vi "H5Tdetect_class.vi"(6 "error in (no error)":errorcluster, 8 "Class":T1 items=["H5T_NO_CLASS"=-1, "H5T_INTEGER"=0, "H5T_FLOAT"=1, "H5T_TIME"=2, "H5T_STRING"=3, "H5T_BITFIELD"=4, "H5T_OPAQUE"=5, "H5T_COMPOUND"=6, "H5T_REFERENCE"=7, "H5T_ENUM"=8, "H5T_VLEN"=9, "H5T_ARRAY"=10], 9 "HDF5 Type Ref":T2) -> (0 "error out":errorcluster, 2 "Detected":bool, 3 "HDF5 Type Ref out":T2)   [LabVIEW 2017]
doc: "Determines whether a datatype contains any datatypes of the \n given datatype class."
uses:
  <vilib>/UPVI/lvhdf5/library.llb/HDF5 Ref.ctl
  <vilib>/UPVI/lvhdf5/datatype.llb/H5T_class_t.ctl
  <vilib>/UPVI/lvhdf5/hdf5.dll
panel:
  # "LVHDF5 Toolkit\nCopyright (c) 2005-2013 by Jason D. Sommerville\nCopyright (c) 2014 by UPVI, LLC.\n\nThis use and distribution of this file is governed by the terms found in \nLICENSE.txt distributed with this toolkit and installed at\n <user.lib>\\_lvhdf5\\LICENSE.txt"
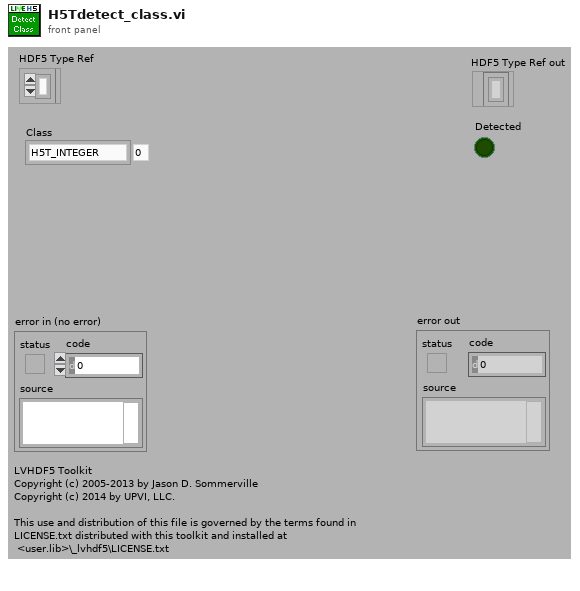
[diagram p1: front panel]
types:
  T1 = typedef "H5T_class_t.ctl" = i32
  T2 = typedef "HDF5 Ref.ctl" = refnum<k1>
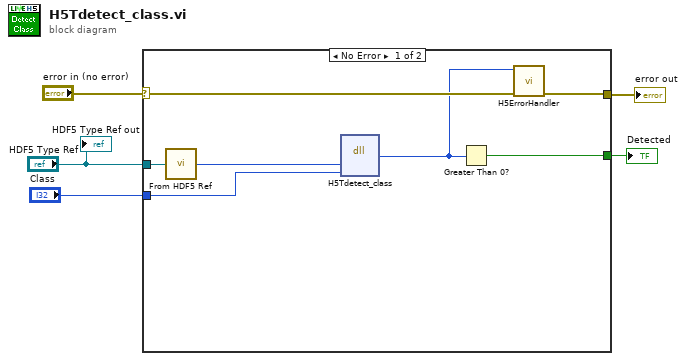
[diagram p0: block diagram]
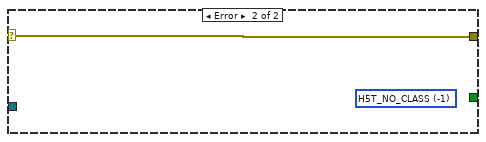
[diagram p2: hidden frame]
diagram:
  n1 = case shown="No Error" "error in (no error)" {
    selector: "error in (no error)" -> [w12 w13]
    tunnel: [w11 w13] -> w4
    tunnel: "HDF5 Type Ref" -> [w10 _]
    tunnel: "Class" -> [w8 _]
    tunnel: [w6 _] -> w1
    frame No Error {
      n2 = call <vilib>:"From HDF5 Ref.vi"("HDF5 Ref"=w10) -> ("I32"=w9:i32)
      n3 = dll-call lib="C:/Program Files/National Instruments/LabVIEW 2017/vi.lib/UPVI/lvhdf5/hdf5.dll" fn="H5Tdetect_class"("type_id"=w9, "dtype_class"=w8) -> ("return type"=w7:i32)  [unwired: 5 in, 2 out]
      n4 = Greater Than 0?(x=w7) -> (x > 0?=w6:bool)
      n5 = call <vilib>:"H5ErrorHandler.vi"("error in (no error)"=w12, "herr_t"=w7) -> ("error out"=w11:errorcluster)  [unwired: 3 in, 4 out]
    }
    frame Error {
      (unwired) -1 items=["H5T_NO_CLASS"=-1, "H5T_INTEGER"=0, "H5T_FLOAT"=1, "H5T_TIME"=2, "H5T_STRING"=3, "H5T_BITFIELD"=4, "H5T_OPAQUE"=5, "H5T_COMPOUND"=6, "H5T_REFERENCE"=7, "H5T_ENUM"=8, "H5T_VLEN"=9, "H5T_ARRAY"=10] ("class")
    }
  }
  "error out" <- w4
  "Detected" <- w1
  "HDF5 Type Ref out" <- "HDF5 Type Ref"
